vi "PAN_TCPSERVER_ClientMngr.vi"(9 "action":T2, 10 "connection":T1, 11 "args":string) -> (1 "Clients":T1[](array[typedef]), 2 "resp":string)   [LabVIEW 2016]
uses:
  private/vis/PAN_TCPSERVER_MngrActionStruct.ctl
  private/vis/PAN_TCPSERVER_ConnectionStruct.ctl
panel:
  in  "udp ref":refnum<k16>
  in  "tcp ref ID":refnum<k5>
  out "ids":string[](array[string])
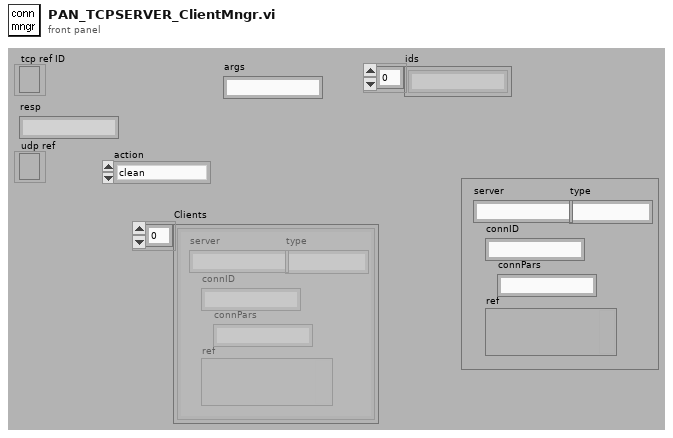
[diagram p1: front panel]
types:
  T1 = typedef "PAN_TCPSERVER_ConnectionStruct.ctl" = cluster{"ref":variant, "connPars":string, "server":string, "connID":string, "type":string}
  T2 = typedef "PAN_TCPSERVER_MngrActionStruct.ctl" = enum16{"clean", "add", "get all", "find by server", "get servers", "delete", "disconnect", "get connection"}
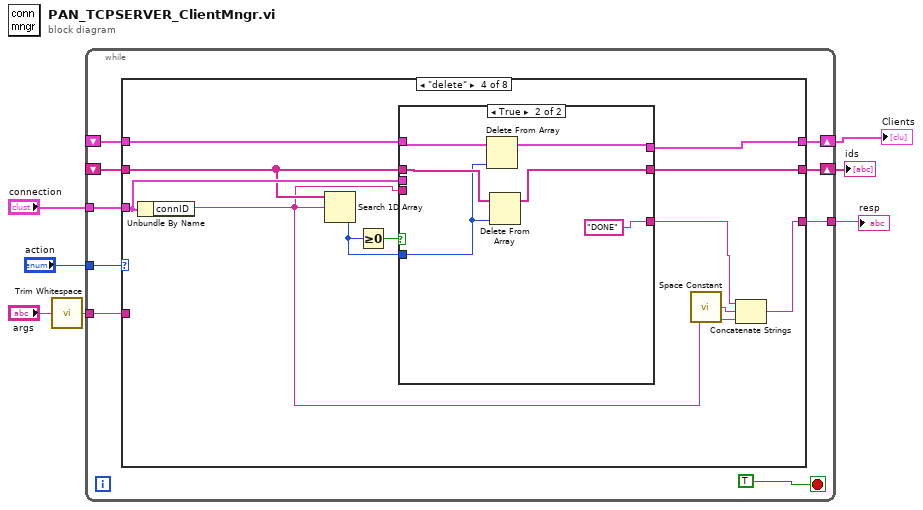
[diagram p0: block diagram]
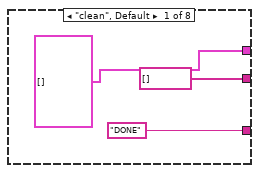
[diagram p2: hidden frame]
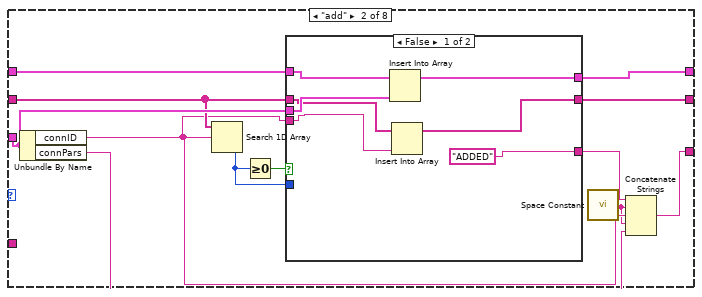
[diagram p3: hidden frame]
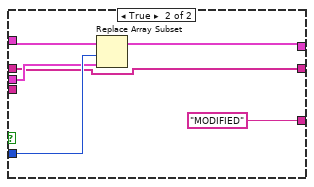
[diagram p4: hidden frame]
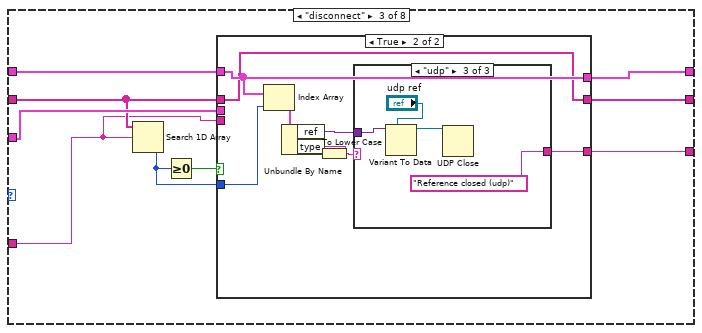
[diagram p5: hidden frame]
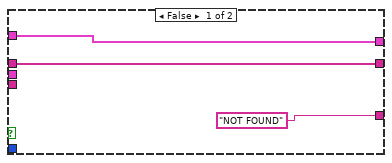
[diagram p6: hidden frame]
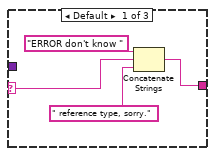
[diagram p7: hidden frame]
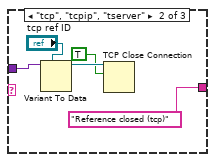
[diagram p8: hidden frame]
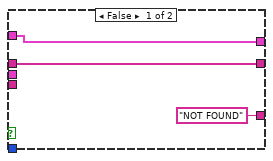
[diagram p9: hidden frame]
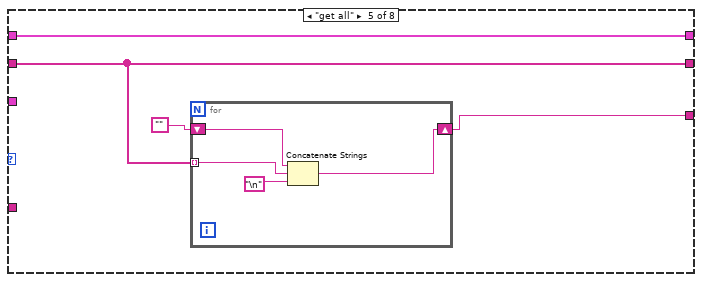
[diagram p10: hidden frame]
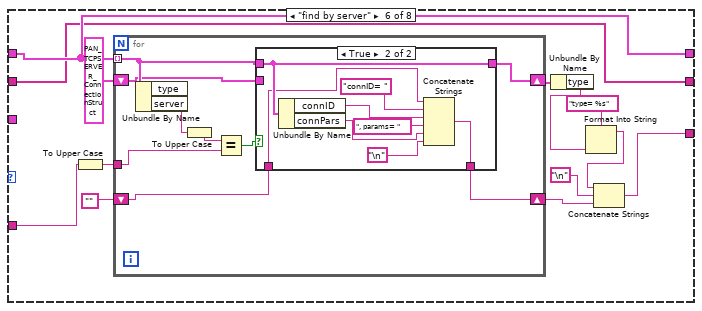
[diagram p11: hidden frame]
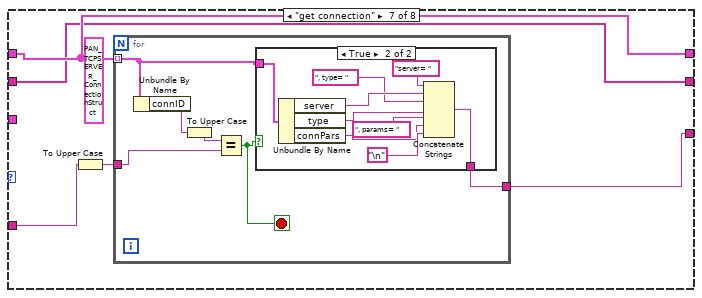
[diagram p13: hidden frame]
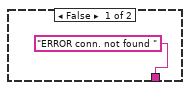
[diagram p14: hidden frame]
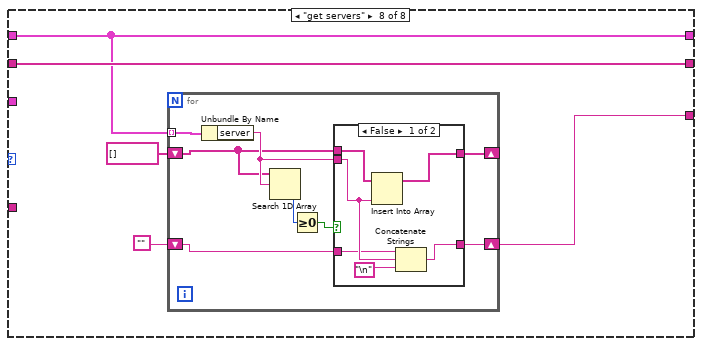
[diagram p15: hidden frame]
diagram:
  n1 = call <vilib>:"Trim Whitespace.vi"("string"="args") -> ("trimmed string"=w1:string)  [unwired: 1 in]
  n2 = while {
    shift-right: [w16] -> w7
    shift-left: _ -> [w15]
    shift-right: [w13] -> w5
    shift-left: _ -> [w12]
    tunnel: "connection" -> [w14]
    tunnel: "action" -> [w11]
    tunnel: [w9] -> w3
    tunnel: w1 -> [w8]
    stop <- TRUE stop-if-true
    n3 = case shown="\"delete\"" w11 {
      tunnel: [T1[] [] ("Clients") w28 w50 w85 w101 w116 w140 w162] -> w16
      tunnel: w15 -> [_ w29 w51 w86 w101 w116 w140 w162]
      tunnel: w14 -> [_ w30 w52 w87 _ _ _ _]
      tunnel: [string[] [] w26 w48 w83 w100 w115 w139 w163] -> w13
      tunnel: w12 -> [_ w25 w46 w82 w100 w115 w139 w163]
      tunnel: ["DONE" ("resp") w22 w47 w80 w99 w106 w138 w161] -> w9
      tunnel: w8 -> [_ _ w45 _ _ w118 w142 _]
      frame "clean", Default {
      }
      frame "add" {
        n4 = Unbundle By Name(w30) -> ("connID"=w23:string, "connPars"=w20:string)
        n5 = Search 1D Array(1D array=w25, element=w23) -> (index of element=w27:i32)  [unwired: 1 out]
        n6 = Greater Or Equal To 0?(x=w27) -> (x >= 0?=w31:bool)
        n7 = case shown="False" w31 {
          tunnel: w30 -> [w36 w42]
          tunnel: w29 -> [w38 w44]
          tunnel: [w37 w41] -> w28
          tunnel: w27 -> [_ w43]
          tunnel: w23 -> [w35 _]
          tunnel: [w34 w40] -> w26
          tunnel: w25 -> [w33 w40]
          tunnel: ["ADDED" ("resp") "MODIFIED" ("resp")] -> w24
          frame False {
            n8 = Insert Into Array(array=w38, new element=w36) -> (w37:T1[])  [unwired: 1 in]
            n9 = Insert Into Array(array=w33, new element=w35) -> (w34:string[])  [unwired: 1 in]
          }
          frame True {
            n10 = Replace Array Subset(array=w44, new element=w42, index=w43) -> (w41:T1[])
          }
        }
        n11 = call <vilib>:"Space Constant.vi"() -> ("String"=w21:string)
        n12 = Concatenate Strings(w24, w21, w23, w21, w20) -> (w22:string)
      }
      frame "disconnect" {
        n13 = Search 1D Array(1D array=w46, element=w45) -> (index of element=w49:i32)  [unwired: 1 out]
        n14 = Greater Or Equal To 0?(x=w49) -> (x >= 0?=w53:bool)
        n15 = case shown="True" w53 {
          tunnel: w52 -> [_ _]
          tunnel: w51 -> [w55 w63]
          tunnel: [w55 w63] -> w50
          tunnel: w49 -> [_ w62]
          tunnel: w45 -> [_ _]
          tunnel: [w54 w57] -> w48
          tunnel: w46 -> [w54 w57]
          tunnel: ["NOT FOUND" ("resp") w64] -> w47
          frame False {
          }
          frame True {
            n16 = Index Array(array=w63, index=w62) -> (element=w61:T1)
            n17 = Unbundle By Name(w61) -> ("ref"=w58:variant, "type"=w60:string)
            n18 = To Lower Case(string=w60) -> (all lower case string=w59:string)
            n19 = case shown="\"udp\"" w59 {
              selector: w59 -> [w67 _ _]
              tunnel: [w65 "Reference closed (tcp)" ("resp") "Reference closed (udp)" ("resp")] -> w64
              tunnel: w58 -> [_ w72 w76]
              frame Default {
                n20 = Concatenate Strings("ERROR don't know " ("string"), w67, " reference type, sorry." ("string")) -> (w65:string)
              }
              frame "tcp", "tcpip", "tserver" {
                n21 = Variant To Data(type="tcp ref ID", Variant=w72) -> (data=w70:refnum<k5>)  [unwired: 1 in, 1 out]
                n22 = TCP Close Connection(connection ID=w70, abort (F)=TRUE) -> ()  [unwired: 1 in, 2 out]
              }
              frame "udp" {
                n23 = Variant To Data(type="udp ref", Variant=w76) -> (data=w74:refnum<k16>)  [unwired: 1 in, 1 out]
                n24 = UDP Close(connection ID=w74) -> ()  [unwired: 1 in, 2 out]
              }
            }
          }
        }
      }
      frame "delete" {
        n25 = Unbundle By Name(w87) -> ("connID"=w78:string)
        n26 = Search 1D Array(1D array=w82, element=w78) -> (index of element=w84:i32)  [unwired: 1 out]
        n27 = Greater Or Equal To 0?(x=w84) -> (x >= 0?=w88:bool)
        n28 = case shown="True" w88 {
          tunnel: w87 -> [_ _]
          tunnel: w86 -> [w91 w97]
          tunnel: [w91 w96] -> w85
          tunnel: w84 -> [_ w93]
          tunnel: w78 -> [_ _]
          tunnel: [w90 w94] -> w83
          tunnel: w82 -> [w90 w95]
          tunnel: ["NOT FOUND" ("resp") "DONE" ("resp")] -> w81
          frame False {
          }
          frame True {
            n29 = Delete From Array(array=w97, index=w93) -> (array with subset deleted=w96:T1[])  [unwired: 1 in, 1 out]
            n30 = Delete From Array(array=w95, index=w93) -> (array with subset deleted=w94:string[])  [unwired: 1 in, 1 out]
          }
        }
        n31 = call <vilib>:"Space Constant.vi"() -> ("String"=w79:string)
        n32 = Concatenate Strings(w81, w79, w78) -> (w80:string)
      }
      frame "get all" {
        n33 = for {
          tunnel: w100 -> [w105] mode=indexing
          shift-right: [w104] -> w99
          shift-left: "" -> [w102]
          n34 = Concatenate Strings(w102, w105, "\n") -> (w104:string)
        }
      }
      frame "find by server" {
        n35 = To Upper Case(1:w118) -> (0:w117:string)
        n36 = for {
          tunnel: w116 -> [w123] mode=indexing
          tunnel: w117 -> [w125]
          shift-right: [w119] -> w107
          shift-left: "" -> [w120]
          shift-right: [w122] -> w111
          shift-left: T1 {"ref"=variant, "connPars"="", "server"="", "connID"="", "type"=""} ("Cluster 2") -> [w121]
          n37 = Unbundle By Name(w123) -> ("server"=w127:string)  [unwired: 1 out]
          n38 = To Upper Case(1:w127) -> (0:w126:string)
          n39 = Equal?(x=w126, y=w125) -> (x = y?=w124:bool)
          n40 = case shown="True" w124 {
            tunnel: w123 -> [_ w132]
            tunnel: [w128 w133] -> w119
            tunnel: [w129 w132] -> w122
            tunnel: w121 -> [w129 _]
            tunnel: w120 -> [w128 w130]
            frame False {
            }
            frame True {
              n41 = Unbundle By Name(w132) -> ("connID"=w136:string, "connPars"=w134:string)
              n42 = Concatenate Strings(w130, "connID= " ("string"), w136, ", params= " ("string"), w134, "\n") -> (w133:string)
            }
          }
        }
        n43 = Unbundle By Name(w111) -> ("type"=w110:string)
        n44 = Format Into String(format string="type= %s", w110) -> (resulting string=w109:string)  [unwired: 2 in, 1 out]
        n45 = Concatenate Strings(w109, "\n", w107) -> (w106:string)
      }
      frame "get connection" {
        (unwired) T1 {"ref"=variant, "connPars"="", "server"="", "connID"="", "type"=""} ("Cluster 2")
        n46 = To Upper Case(1:w142) -> (0:w141:string)
        n47 = for {
          tunnel: w140 -> [w145] mode=indexing
          tunnel: w141 -> [w146]
          tunnel: [w144] -> w138
          stop <- w143 stop-if-true
          n48 = Unbundle By Name(w145) -> ("connID"=w148:string)
          n49 = To Upper Case(1:w148) -> (0:w147:string)
          n50 = Equal?(x=w147, y=w146) -> (x = y?=w143:bool)
          n51 = case shown="True" w143 {
            tunnel: w145 -> [_ w156]
            tunnel: ["ERROR conn. not found " w157] -> w144
            frame False {
            }
            frame True {
              n52 = Unbundle By Name(w156) -> ("server"=w153:string, "type"=w150:string, "connPars"=w152:string)
              n53 = Concatenate Strings("server= " ("string"), w153, ", type= " ("string"), w150, ", params= " ("string"), w152, "\n") -> (w157:string)
            }
          }
        }
      }
      frame "get servers" {
        n54 = for {
          tunnel: w162 -> [w171] mode=indexing
          shift-right: [w167] -> _
          shift-left: string[] [] -> [w164]
          shift-right: [w166] -> w161
          shift-left: "" -> [w165]
          n55 = Unbundle By Name(w171) -> ("server"=w168:string)
          n56 = Search 1D Array(1D array=w164, element=w168) -> (index of element=w170:i32)  [unwired: 1 out]
          n57 = Greater Or Equal To 0?(x=w170) -> (x >= 0?=w169:bool)
          n58 = case shown="False" w169 {
            tunnel: w168 -> [w175 _]
            tunnel: [w177 w179] -> w167
            tunnel: w164 -> [w176 w179]
            tunnel: [w174 w178] -> w166
            tunnel: w165 -> [w173 w178]
            frame False {
              n59 = Insert Into Array(array=w176, new element=w175) -> (w177:string[])  [unwired: 1 in]
              n60 = Concatenate Strings(w173, w175, "\n") -> (w174:string)
            }
            frame True {
            }
          }
        }
      }
    }
  }
  "Clients" <- w7
  "ids" <- w5
  "resp" <- w3
